vi "RetaInimigoBolaUsandoOrientacao.vi"(4 "Goal Width":u32, 5 "Field length":u32, 7 "Meio?":bool=TRUE, 8 "Orientação inimigo":dbl format="%#_13g", 10 "Y bola":dbl format="%#_13g", 11 "X bola":dbl format="%#_13g") -> (1 "Orientação goleiro":dbl format="%#_13g", 2 "Y golerio":dbl format="%#_13g", 3 "X goleiro":dbl format="%#_13g")   [LabVIEW 2017]
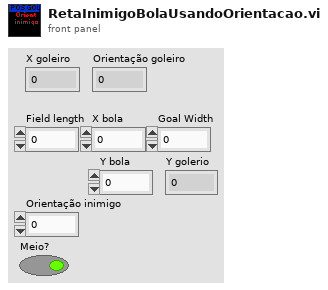
[diagram p1: front panel]
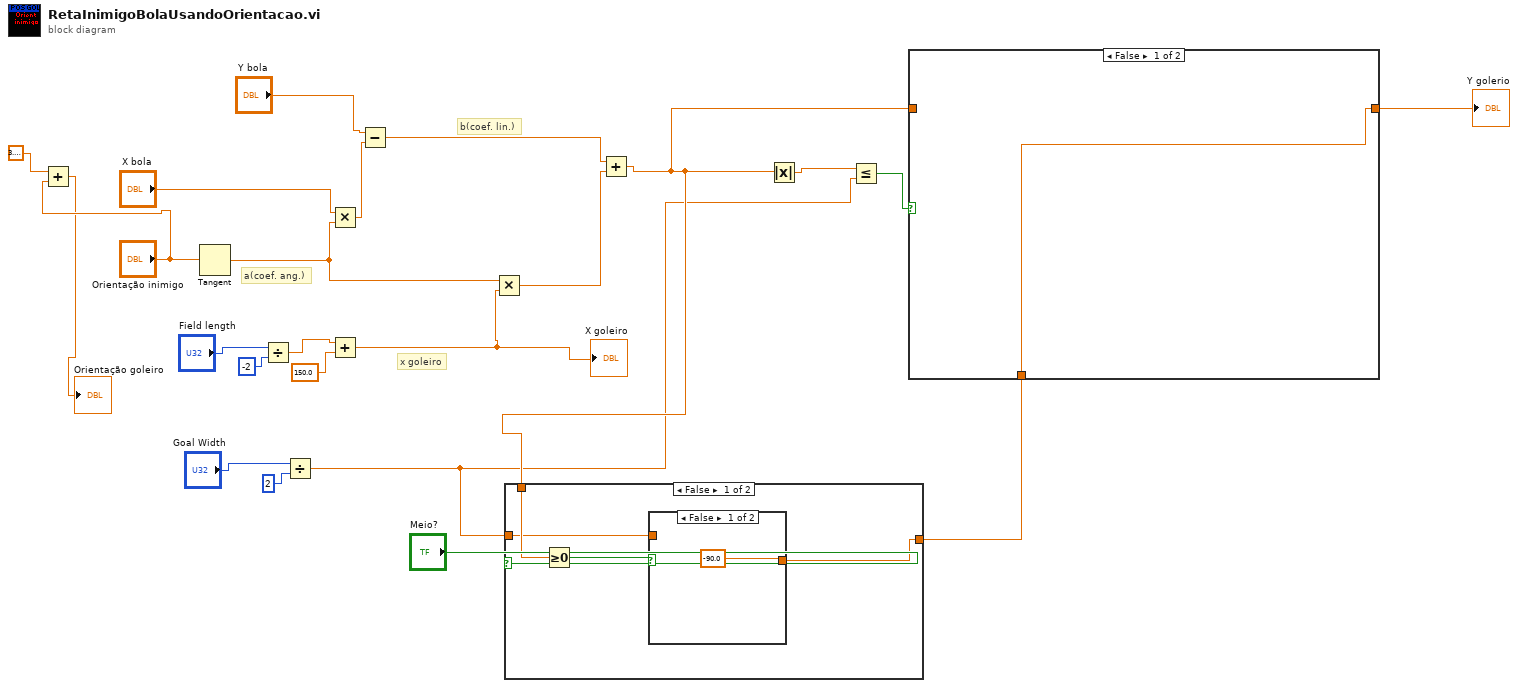
[diagram p0: block diagram]
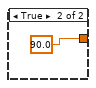
[diagram p2: hidden frame]
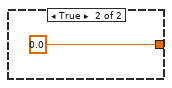
[diagram p3: hidden frame]
diagram:
  # "b(coef. lin.)"
  # "x goleiro"
  # "a(coef. ang.)"
  n1 = Add(x=3.141592653589793, y="Orientação inimigo") -> (x+y=→"Orientação goleiro":dbl)
  n2 = Tangent(1:"Orientação inimigo") -> (0:w16:dbl)
  n3 = Divide(x="Field length", y=-2) -> (x/y=w18:dbl)
  n4 = Divide(x="Goal Width", y=2) -> (x/y=w5:dbl)
  n5 = Multiply(x="X bola", y=w16) -> (x*y=w21:dbl)
  n6 = Add(x=w18, y=150.0 ("x+y")) -> (x+y=w1:dbl)
  "X goleiro" <- w1
  n7 = Subtract(x="Y bola", y=w21) -> (x-y=w15:dbl)
  n8 = Multiply(x=w16, y=w1) -> (x*y=w14:dbl)
  n9 = Add(x=w15, y=w14) -> (x+y=w6:dbl)
  n10 = case shown="False" "Meio?" {
    tunnel: [w24 0.0] -> w7
    tunnel: w6 -> [w27 _]
    tunnel: w5 -> [w25 _]
    frame False {
      n11 = Greater Or Equal To 0?(x=w27) -> (x >= 0?=w26:bool)
      n12 = case shown="False" w26 {
        tunnel: w25 -> [_ _]
        tunnel: [-90.0 ("y") 90.0 ("y")] -> w24
        frame False {
        }
        frame True {
        }
      }
    }
    frame True {
    }
  }
  n13 = Absolute Value(x=w6) -> (abs(x)=w11:dbl)
  n14 = Less Or Equal?(x=w11, y=w5) -> (x <= y?=w10:bool)
  n15 = case shown="False" w10 {
    tunnel: [w31 w32] -> w8
    tunnel: w6 -> [_ w32]
    tunnel: w7 -> [w31 _]
    frame False {
    }
    frame True {
    }
  }
  "Y golerio" <- w8
